vi "Mecanum.vi"(3 "Low Speed Mode":bool, 4 "Controller Type":T1=enum."Xbox 360", 5 "Joystick Values":dbl[](array[numeric])) -> (0 "Spin":dbl, 1 "Y Setpoint":dbl, 2 "X Setpoint":dbl)   [LabVIEW 2016]
uses:
  Joystick Types.ctl
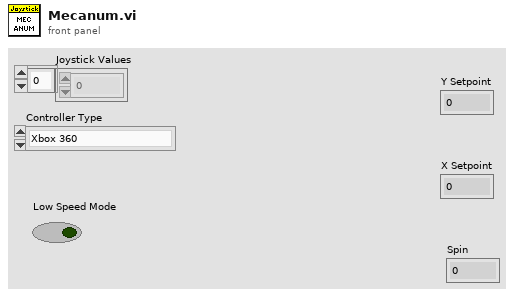
[diagram p1: front panel]
types:
  T1 = typedef "Joystick Types.ctl" = enum16{"Extreme 3D Pro", "Xbox 360"}
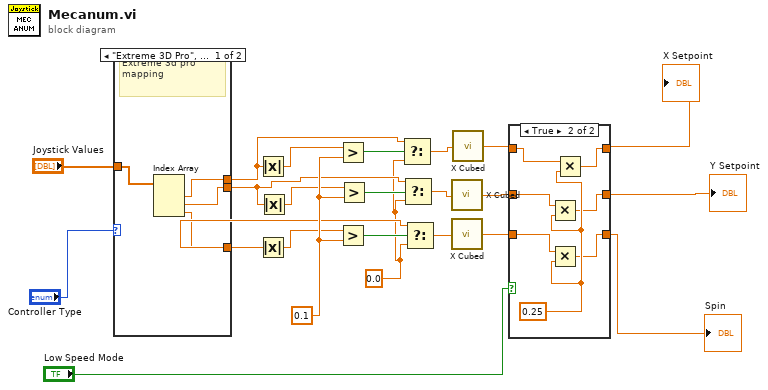
[diagram p0: block diagram]
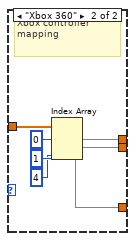
[diagram p2: hidden frame]
diagram:
  w12 = 0.0
  w19 = 0.1
  n1 = case shown="\"Extreme 3D Pro\", Default" "Controller Type" {
    tunnel: "Joystick Values" -> [w27 w34]
    tunnel: [w26 w30] -> w15
    tunnel: [w25 w29] -> w14
    tunnel: [w24 w28] -> w13
    frame "Extreme 3D Pro", Default {
      # "Extreme 3d pro \nmapping"
      n2 = Index Array(array=w27) -> (element #1=w26:dbl, element #2=w25:dbl, element #3=w24:dbl)  [unwired: 3 in]
    }
    frame "Xbox 360" {
      # "Xbox controller\nmapping"
      n3 = Index Array(array=w34, index #1=0 ("index"), index #2=1 ("index"), index #3=4 ("index")) -> (element #1=w30:dbl, element #2=w29:dbl, element #3=w28:dbl)
    }
  }
  n4 = Absolute Value(x=w15) -> (abs(x)=w18:dbl)
  n5 = Absolute Value(x=w13) -> (abs(x)=w16:dbl)
  n6 = Absolute Value(x=w14) -> (abs(x)=w17:dbl)
  n7 = Greater?(x=w18, y=w19) -> (0:w22:bool)
  n8 = Greater?(x=w16, y=w19) -> (0:w20:bool)
  n9 = Greater?(x=w17, y=w19) -> (0:w21:bool)
  n10 = Select(t=w15, s=w22, f=w12) -> (s? t:f=w11:dbl)
  n11 = Select(t=w14, s=w21, f=w12) -> (s? t:f=w10:dbl)
  n12 = Select(t=w13, s=w20, f=w12) -> (s? t:f=w9:dbl)
  n13 = call "X Cubed.vi"("X"=w10) -> ("X^3"=w5:dbl)
  n14 = call "X Cubed.vi"("X"=w9) -> ("X^3"=w4:dbl)
  n15 = call "X Cubed.vi"("X"=w11) -> ("X^3"=w6:dbl)
  n16 = case shown="True" "Low Speed Mode" {
    tunnel: w6 -> [w35 w42]
    tunnel: w5 -> [w36 w43]
    tunnel: w4 -> [w37 w44]
    tunnel: [w37 w39] -> w3
    tunnel: [w36 w40] -> w2
    tunnel: [w35 w38] -> w1
    frame False {
    }
    frame True {
      w41 = 0.25
      n17 = Multiply(x=w43, y=w41) -> (x*y=w40:dbl)
      n18 = Multiply(x=w44, y=w41) -> (x*y=w39:dbl)
      n19 = Multiply(x=w42, y=w41) -> (x*y=w38:dbl)
    }
  }
  "Y Setpoint" <- w2
  "X Setpoint" <- w1
  "Spin" <- w3
